vi "Differential Pressure Release Valve Test.vi"(8 "error in (no error)":errorcluster, 10 "Model in":refnum<class "Model.lvclass">, 11 "Test Actuator State in":refnum<class "Test Actuator State.lvclass">) -> (0 "error out":errorcluster, 2 "Model out":refnum<class "Model.lvclass">, 3 "Test Actuator State out":refnum<class "Test Actuator State.lvclass">)   [LabVIEW 2016, in "Test Actuator State.lvclass"]
uses:
  Test Actuator State.lvclass
  Model/Model/Model.lvclass
  Typedefs/TestStatus.ctl
  Model/Model/Model.lvclass/Model.ctl
  Typedefs/FAMT Typedefs.lvlib
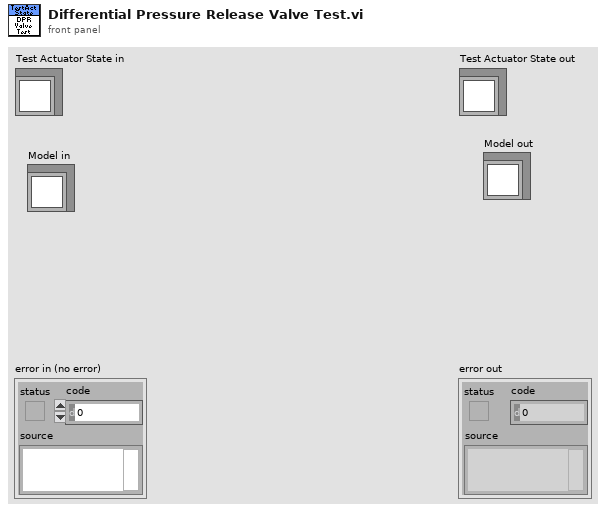
[diagram p1: front panel]
types:
  T1 = typedef "FAMT Typedefs.lvlib/TestStatus.ctl" = enum16{"Not Run", "Running", "Passed", "Failed"}
  T2 = typedef "FAMT Typedefs.lvlib/AllTestStatus.ctl" = cluster{"Differential Pressure Release Valve Test":T1, "Force Accuracy Test":T1, "Full Force Test":T1, "Operational Force Test":T1, "Sentran Accuracy Test":T1, "Slewing Test":T1, "Tracking Test":T1}
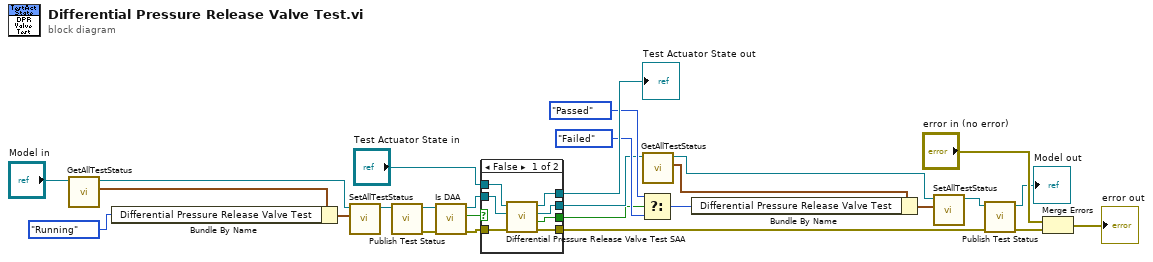
[diagram p0: block diagram]
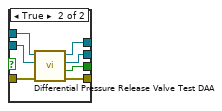
[diagram p2: hidden frame]
diagram:
  n1 = call "GetAllTestStatus.vi"("Model in"="Model in") -> ("AllTestStatus"=w16:T2, "Model out"=w19:refnum<class "Model.lvclass">)  [unwired: 9 in]
  n2 = Bundle By Name(cluster=w16, "Differential Pressure Release Valve Test"=TestStatus."Running" ("Full Force Test")) -> (w17:T2)
  n3 = call "SetAllTestStatus.vi"("AllTestStatus"=w17, "Model in"=w19) -> ("Model out"=w20:refnum<class "Model.lvclass">)  [unwired: 9 in]
  n4 = call "Publish Test Status.vi"("Model in"=w20) -> ("error out"=w13:errorcluster, "Model out"=w14:refnum<class "Model.lvclass">)  [unwired: 9 in]
  n5 = call "Is DAA.vi"("error in (no error)"=w13, "Model in"=w14) -> ("error out"=w23:errorcluster, "IsDAA"=w25:bool, "Model out"=w22:refnum<class "Model.lvclass">)  [unwired: 7 in]
  n6 = case shown="False" w25 {
    tunnel: "Test Actuator State in" -> [w34 w41]
    tunnel: w23 -> [w30 w38]
    tunnel: w22 -> [w32 w39]
    tunnel: [w33 w40] -> w21
    tunnel: [w31 w36] -> w5
    tunnel: [w29 w37] -> w4
    tunnel: [w28 w35] -> w3
    frame False {
      n7 = call "Differential Pressure Release Valve Test SAA.vi"("error in (no error)"=w30, "Model in"=w32, "Test Actuator State in"=w34) -> ("error out"=w29:errorcluster, "Pass"=w28:bool, "Model out"=w31:refnum<class "Model.lvclass">, "Test Actuator State out"=w33:refnum<class "Test Actuator State.lvclass">)  [unwired: 5 in]
    }
    frame True {
      n8 = call "Differential Pressure Release Valve Test DAA.vi"("error in (no error)"=w38, "Model in"=w39, "Test Actuator State in"=w41) -> ("error out"=w37:errorcluster, "Pass"=w35:bool, "Model out"=w36:refnum<class "Model.lvclass">, "Test Actuator State out"=w40:refnum<class "Test Actuator State.lvclass">)  [unwired: 5 in]
    }
  }
  "Test Actuator State out" <- w21
  n9 = Select(t=TestStatus."Passed" ("Full Force Test"), s=w3, f=TestStatus."Failed" ("Full Force Test")) -> (s? t:f=w8:T1)
  n10 = call "GetAllTestStatus.vi"("Model in"=w5) -> ("AllTestStatus"=w12:T2, "Model out"=w10:refnum<class "Model.lvclass">)  [unwired: 9 in]
  n11 = Bundle By Name(cluster=w12, "Differential Pressure Release Valve Test"=w8) -> (w11:T2)
  n12 = call "SetAllTestStatus.vi"("AllTestStatus"=w11, "Model in"=w10) -> ("Model out"=w9:refnum<class "Model.lvclass">)  [unwired: 9 in]
  n13 = call "Publish Test Status.vi"("error in (no error)"=w4, "Model in"=w9) -> ("error out"=w1:errorcluster, "Model out"=→"Model out":refnum<class "Model.lvclass">)  [unwired: 8 in]
  n14 = Merge Errors("error in (no error)", w1) -> (→"error out":errorcluster)
